vi "Drive Distance (Inches).vi"(8 "Right Speed":dbl=0.8 format="%#_13g", 9 "Left Speed":dbl=0.8 format="%#_13g", 10 "inches":dbl format="%#_13g") -> ()   [LabVIEW 2015]
uses:
  Sprocket/src/Action/Action Name.ctl
  Drive/Drive States.ctl
  Sprocket/src/Refname/Refname to String.vi
  Sprocket/src/Refname/Refname to String (Queue).vi
  Sprocket/src/Stream/Obtain Stream.vi
  Sprocket/src/Stream/Push Stream.vi
  Sprocket/src/Stream/Release Stream.vi
  Main/Robot Global Data.vi
  Sprocket/lib/Sprocket.lvlib
panel:
  in  "Q":dbl=0.93
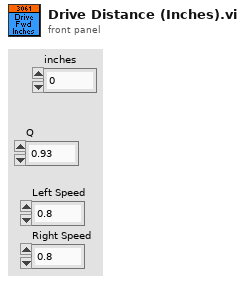
[diagram p1: front panel]
types:
  T1 = typedef "Sprocket.lvlib/Action Name.ctl" = enum16{"No Action", "Drive Train Both", "Drive Train Rotate", "Drive Train Throttle", "Collector Motor Roll", "Collector Motor Eject", "Collector Motor Collect", "Collector Motor Stop", "Collector Extend", "Collector Retract", "Shifter High", "Shifter Low", "Collector Motor Stall", "Wedge Roll"}
  T2 = typedef "Drive States.ctl" = enum16{"Idle", "Teleop", "Start Rotate", "Do Rotate", "Stop Rotate", "Start Throttle", "Do Throttle", "Stop Throttle"}
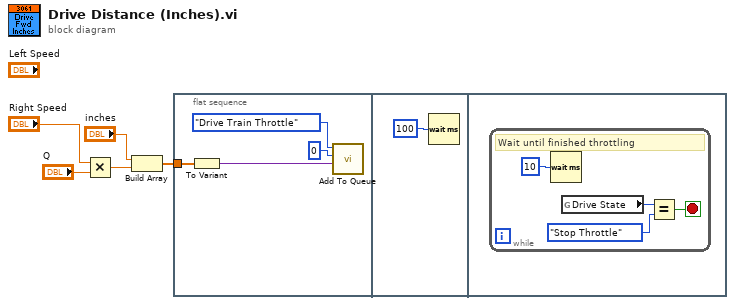
[diagram p0: block diagram]
diagram:
  n1 = Multiply(x="Right Speed", y="Q") -> (x*y=w2:dbl)
  n2 = Build Array("inches", w2) -> (w3:dbl[])
  n3 = flat-sequence {
    tunnel: w3 -> [w6]
    frame #0 {
      n4 = To Variant(anything=w6) -> (Variant=w7:variant)
      n5 = call "Add To Queue.vi"("Data"=w7, "Priority"=0, "Action"=Action_Name."Drive Train Throttle") -> ()  [unwired: 8 in, 1 out]
    }
    frame #1 {
      n6 = Wait (ms)(milliseconds to wait=u32 100) -> ()  [unwired: 1 out]
    }
    frame #2 {
      n7 = while {
        stop <- w13 stop-if-true
        # "Wait until finished throttling"
        n8 = Wait (ms)(milliseconds to wait=u32 10) -> ()  [unwired: 1 out]
        n9 = global read "Robot Global Data.vi" "Drive State"() -> (w14:T2)
        n10 = Equal?(x=w14, y=Drive_States."Stop Throttle" ("t")) -> (x = y?=w13:bool)
      }
    }
  }
